vi "young2.vi"() -> ()   [LabVIEW 2011]
uses:
  <instrlib>/Tektronix DPO MSO 2000 4000 Series/Public/Data/Read (Multiple Waveforms).vi
  <vilib>/express/express analysis/Spectral/Block/exnSpectralBlock spectral measurements RMS poly.vi
  <vilib>/express/express analysis/Spectral/Block/exnSpectralBlock spectral measurements RMS array WFM.vi
  <vilib>/express/express analysis/Spectral/XNode/ExpressSpectralMeasurementsBlockNode.xnode
  <instrlib>/Tektronix DPO MSO 2000 4000 Series/Tektronix DPO MSO 2000 4000 Series.lvlib
panel:
  in  "?":bool
  out "Channel 2 FFT":cluster{"f0":dbl, "df":dbl, "magnitude":dbl[]}[](graph)
  out "Channel 2":waveform(dbl)[](graph)
  out "Channel1 FFT":cluster{"f0":dbl, "df":dbl, "magnitude":dbl[]}[](graph)
  out "Channel 1":waveform(dbl)[](graph)
  in  "VISA resource name":refnum<visa-resource-name>
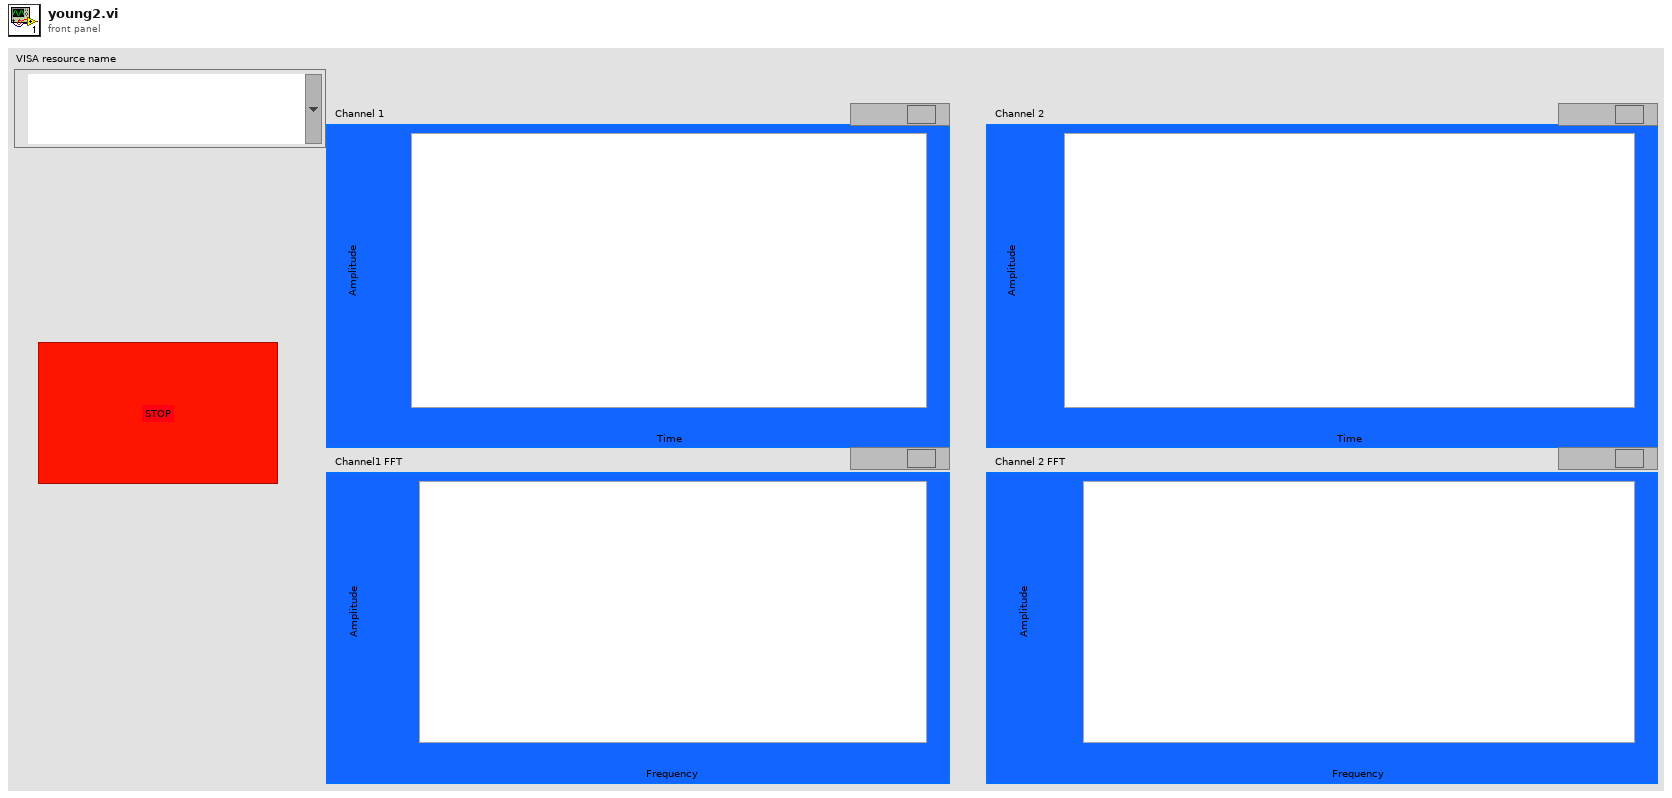
[diagram p1: front panel]
types:
  T1 = cluster{"averaging mode":u16, "weighting mode":u16, "number of averages":u32}
  T2 = cluster{"dB On (F)":bool, "unwrap phase (F)":bool, "convert to degree (F)":bool}
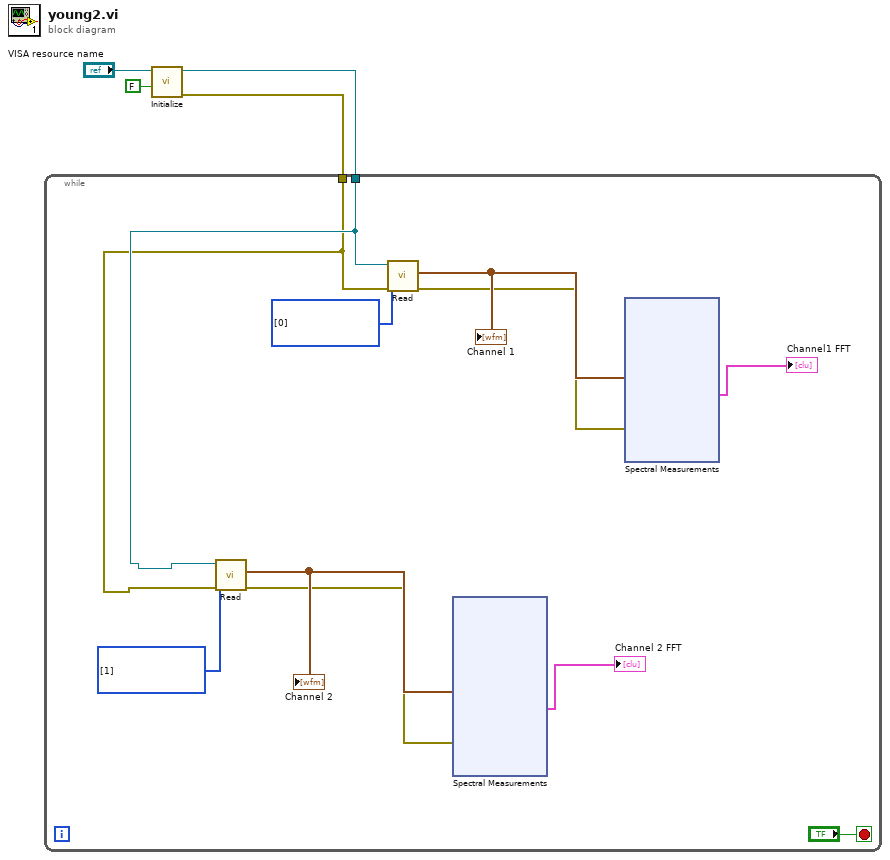
[diagram p0: block diagram]
diagram:
  n1 = call <instrlib>:"Initialize.vi"("Reset (True)"=FALSE, "VISA resource name"="VISA resource name") -> ("error out"=w1:errorcluster, "VISA resource name out"=w2:refnum<visa-resource-name>)  [unwired: 8 in]
  n2 = while {
    tunnel: w2 -> [w7]
    tunnel: w1 -> [w6]
    stop <- "?" stop-if-true
    w8 = u16[] [1] items=["Channel 1", "Channel 2", "Channel 3", "Channel 4", "Math", "Reference 1", "Reference 2", "Reference 3", "Reference 4"] ("Channels")
    w12 = u16[] [0] items=["Channel 1", "Channel 2", "Channel 3", "Channel 4", "Math", "Reference 1", "Reference 2", "Reference 3", "Reference 4"] ("Channels")
    n3 = call-poly <instrlib>:"Read.vi"("error in (no error)"=w6, "Channels"=w8, "VISA resource name"=w7) -> ("error out"=w10:errorcluster, "Waveform Data"=w11:waveform(dbl)[])  [unwired: 6 in, 1 out]
    "Channel 2" <- w11
    n4 = call-poly <instrlib>:"Read.vi"("error in (no error)"=w6, "Channels"=w12, "VISA resource name"=w7) -> ("error out"=w14:errorcluster, "Waveform Data"=w15:waveform(dbl)[])  [unwired: 6 in, 1 out]
    "Channel 1" <- w15
    n5 = xnode "Spectral Measurements"("Signals"=w11, "error in (no error)"=w10) -> ("FFT - (RMS)"=→"Channel 2 FFT":cluster{"f0":dbl, "df":dbl, "magnitude":dbl[]}[])  [unwired: 2 out]
    n6 = xnode "Spectral Measurements"("Signals"=w15, "error in (no error)"=w14) -> ("FFT - (RMS)"=→"Channel1 FFT":cluster{"f0":dbl, "df":dbl, "magnitude":dbl[]}[])  [unwired: 2 out]
  }
